vi "Init.vi"(8 "error in (no error)":errorcluster, 11 "Fgen VISA CFG in":refnum<class "Fgen VISA CFG.lvclass">) -> (0 "error out":errorcluster, 3 "Fgen VISA CFG out":refnum<class "Fgen VISA CFG.lvclass">)   [LabVIEW 2023, in "Fgen VISA CFG.lvclass"]
uses:
  Fgen VISA CFG.lvclass
  Fgen VISA CFG.lvclass/Fgen VISA CFG.ctl
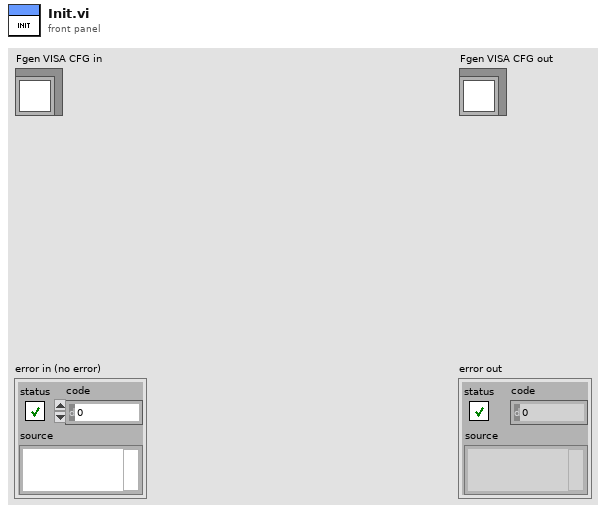
[diagram p1: front panel]
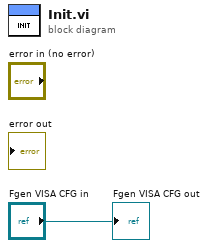
[diagram p0: block diagram]
diagram:
  "Fgen VISA CFG out" <- "Fgen VISA CFG in"
